vi "MeasureGrowth.vi"(10 "DaysBack":i32=7, 11 "Data":cluster{"Cases":i32[], "Days":timestamp[]}={"Cases"=[0, 0, 0, 0, 2, 2, 2, 2, 2, 3, 3, 3, 6, 6, 6, 6, 6, 6, 6, 6, 7, 7, 8, 8, 8, 8, 8, 8, 8, 8, 10, 10, 10, 10, 10, 10, 11, 11, 12, 12, 21, 25, 35, 51, 59, 102, 116, 167, 179, 247, 250, 305, 372, 480, 588, 741, 892, 1065, 1289, 1524, 1826, 2253, 2641, 3176, 4035, 4863, 5671, 6352, 7412, 8570, 9939, 11170, 12563, 13886], "Days"=[timestamp(3662524800 s since 1904-01-01), timestamp(3662611200 s since 1904-01-01), timestamp(3662697600 s since 1904-01-01), timestamp(3662784000 s since 1904-01-01), timestamp(3662870400 s since 1904-01-01), timestamp(3662956800 s since 1904-01-01), timestamp(3663043200 s since 1904-01-01), timestamp(3663129600 s since 1904-01-01), timestamp(3663216000 s since 1904-01-01), timestamp(3663302400 s since 1904-01-01), timestamp(3663388800 s since 1904-01-01), timestamp(3663475200 s since 1904-01-01), timestamp(3663561600 s since 1904-01-01), timestamp(3663648000 s since 1904-01-01), timestamp(3663734400 s since 1904-01-01), timestamp(3663820800 s since 1904-01-01), timestamp(3663907200 s since 1904-01-01), timestamp(3663993600 s since 1904-01-01), timestamp(3664080000 s since 1904-01-01), timestamp(3664166400 s since 1904-01-01), timestamp(3664252800 s since 1904-01-01), timestamp(3664339200 s since 1904-01-01), timestamp(3664425600 s since 1904-01-01), timestamp(3664512000 s since 1904-01-01), timestamp(3664598400 s since 1904-01-01), timestamp(3664684800 s since 1904-01-01), timestamp(3664771200 s since 1904-01-01), timestamp(3664857600 s since 1904-01-01), timestamp(3664944000 s since 1904-01-01), timestamp(3665030400 s since 1904-01-01), timestamp(3665116800 s since 1904-01-01), timestamp(3665203200 s since 1904-01-01), timestamp(3665289600 s since 1904-01-01), timestamp(3665376000 s since 1904-01-01), timestamp(3665462400 s since 1904-01-01), timestamp(3665548800 s since 1904-01-01), timestamp(3665635200 s since 1904-01-01), timestamp(3665721600 s since 1904-01-01), timestamp(3665808000 s since 1904-01-01), timestamp(3665894400 s since 1904-01-01), timestamp(3665980800 s since 1904-01-01), timestamp(3666067200 s since 1904-01-01), timestamp(3666153600 s since 1904-01-01), timestamp(3666240000 s since 1904-01-01), timestamp(3666326400 s since 1904-01-01), timestamp(3666412800 s since 1904-01-01), timestamp(3666499200 s since 1904-01-01), timestamp(3666585600 s since 1904-01-01), timestamp(3666672000 s since 1904-01-01), timestamp(3666758400 s since 1904-01-01), timestamp(3666844800 s since 1904-01-01), timestamp(3666931200 s since 1904-01-01), timestamp(3667017600 s since 1904-01-01), timestamp(3667104000 s since 1904-01-01), timestamp(3667190400 s since 1904-01-01), timestamp(3667276800 s since 1904-01-01), timestamp(3667363200 s since 1904-01-01), timestamp(3667449600 s since 1904-01-01), timestamp(3667536000 s since 1904-01-01), timestamp(3667622400 s since 1904-01-01), timestamp(3667708800 s since 1904-01-01), timestamp(3667795200 s since 1904-01-01), timestamp(3667881600 s since 1904-01-01), timestamp(3667968000 s since 1904-01-01), timestamp(3668054400 s since 1904-01-01), timestamp(3668140800 s since 1904-01-01), timestamp(3668227200 s since 1904-01-01), timestamp(3668313600 s since 1904-01-01), timestamp(3668400000 s since 1904-01-01), timestamp(3668486400 s since 1904-01-01), timestamp(3668572800 s since 1904-01-01), timestamp(3668659200 s since 1904-01-01), timestamp(3668745600 s since 1904-01-01), timestamp(3668832000 s since 1904-01-01)]}) -> (0 "Plot":T1(graph)=[{"Days"=[timestamp(3662524800 s since 1904-01-01), timestamp(3662611200 s since 1904-01-01), timestamp(3662697600 s since 1904-01-01), timestamp(3662784000 s since 1904-01-01), timestamp(3662870400 s since 1904-01-01), timestamp(3662956800 s since 1904-01-01), timestamp(3663043200 s since 1904-01-01), timestamp(3663129600 s since 1904-01-01), timestamp(3663216000 s since 1904-01-01), timestamp(3663302400 s since 1904-01-01), timestamp(3663388800 s since 1904-01-01), timestamp(3663475200 s since 1904-01-01), timestamp(3663561600 s since 1904-01-01), timestamp(3663648000 s since 1904-01-01), timestamp(3663734400 s since 1904-01-01), timestamp(3663820800 s since 1904-01-01), timestamp(3663907200 s since 1904-01-01), timestamp(3663993600 s since 1904-01-01), timestamp(3664080000 s since 1904-01-01), timestamp(3664166400 s since 1904-01-01), timestamp(3664252800 s since 1904-01-01), timestamp(3664339200 s since 1904-01-01), timestamp(3664425600 s since 1904-01-01), timestamp(3664512000 s since 1904-01-01), timestamp(3664598400 s since 1904-01-01), timestamp(3664684800 s since 1904-01-01), timestamp(3664771200 s since 1904-01-01), timestamp(3664857600 s since 1904-01-01), timestamp(3664944000 s since 1904-01-01), timestamp(3665030400 s since 1904-01-01), timestamp(3665116800 s since 1904-01-01), timestamp(3665203200 s since 1904-01-01), timestamp(3665289600 s since 1904-01-01), timestamp(3665376000 s since 1904-01-01), timestamp(3665462400 s since 1904-01-01), timestamp(3665548800 s since 1904-01-01), timestamp(3665635200 s since 1904-01-01), timestamp(3665721600 s since 1904-01-01), timestamp(3665808000 s since 1904-01-01), timestamp(3665894400 s since 1904-01-01), timestamp(3665980800 s since 1904-01-01), timestamp(3666067200 s since 1904-01-01), timestamp(3666153600 s since 1904-01-01), timestamp(3666240000 s since 1904-01-01), timestamp(3666326400 s since 1904-01-01), timestamp(3666412800 s since 1904-01-01), timestamp(3666499200 s since 1904-01-01), timestamp(3666585600 s since 1904-01-01), timestamp(3666672000 s since 1904-01-01), timestamp(3666758400 s since 1904-01-01), timestamp(3666844800 s since 1904-01-01), timestamp(3666931200 s since 1904-01-01), timestamp(3667017600 s since 1904-01-01), timestamp(3667104000 s since 1904-01-01), timestamp(3667190400 s since 1904-01-01), timestamp(3667276800 s since 1904-01-01), timestamp(3667363200 s since 1904-01-01), timestamp(3667449600 s since 1904-01-01), timestamp(3667536000 s since 1904-01-01), timestamp(3667622400 s since 1904-01-01), timestamp(3667708800 s since 1904-01-01), timestamp(3667795200 s since 1904-01-01), timestamp(3667881600 s since 1904-01-01), timestamp(3667968000 s since 1904-01-01), timestamp(3668054400 s since 1904-01-01), timestamp(3668140800 s since 1904-01-01), timestamp(3668227200 s since 1904-01-01), timestamp(3668313600 s since 1904-01-01), timestamp(3668400000 s since 1904-01-01), timestamp(3668486400 s since 1904-01-01), timestamp(3668572800 s since 1904-01-01), timestamp(3668659200 s since 1904-01-01), timestamp(3668745600 s since 1904-01-01), timestamp(3668832000 s since 1904-01-01)], "ConfirmedCases"=[0.0, 0.0, 0.0, 0.0, 0.0, 0.0, 0.0, 0.0, 0.0, 0.0, 0.0, 0.0, 0.0, 0.0, 0.0, 0.0, 0.0, 0.0, 0.0, 0.0, 0.0, 0.0, 0.0, 0.0, 0.0, 0.0, 0.0, 0.0, 0.0, 0.0, 0.0, 0.0, 0.0, 0.0, 0.0, 0.0, 0.0, 0.0, 0.0, 0.0, 0.0, 0.0, 1.0, 1.0, 1.0, 1.0, 1.0, 2.0, 3.0, 4.0, 4.0, 4.0, 4.0, 6.0, 11.0, 14.0, 17.0, 19.0, 24.0, 29.0, 33.0, 40.0, 52.0, 67.0, 83.0, 100.0, 121.0, 132.0, 149.0, 182.0, 212.0, 243.0, 282.0, 321.0]}, {"Days"=[timestamp(3668313600 s since 1904-01-01), timestamp(3668400000 s since 1904-01-01), timestamp(3668486400 s since 1904-01-01), timestamp(3668572800 s since 1904-01-01), timestamp(3668659200 s since 1904-01-01), timestamp(3668745600 s since 1904-01-01), timestamp(3668832000 s since 1904-01-01)], "ConfirmedCases"=[132.01823524302534, 153.55263572024907, 178.59966006386384, 207.73227646213113, 241.6169138771523, 281.0287070731711, 326.8692283660796]}, {"Days"=[timestamp(3668313600 s since 1904-01-01), timestamp(3668400000 s since 1904-01-01), timestamp(3668486400 s since 1904-01-01), timestamp(3668572800 s since 1904-01-01), timestamp(3668659200 s since 1904-01-01), timestamp(3668745600 s since 1904-01-01), timestamp(3668832000 s since 1904-01-01)], "ConfirmedCases"=[140.59609548662908, 162.8828644131387, 188.9766356577397, 219.6124606618654, 255.65531024069676, 298.10468948116306, 348.1074955925532]}, {"Days"=[timestamp(3668313600 s since 1904-01-01), timestamp(3668400000 s since 1904-01-01), timestamp(3668486400 s since 1904-01-01), timestamp(3668572800 s since 1904-01-01), timestamp(3668659200 s since 1904-01-01), timestamp(3668745600 s since 1904-01-01), timestamp(3668832000 s since 1904-01-01)], "ConfirmedCases"=[123.96371589380509, 144.75685960943596, 168.7924989452066, 196.49476425010758, 228.34938580605382, 264.9308682016178, 306.9267217896756]}, {"Days"=[timestamp(3668313600 s since 1904-01-01), timestamp(3668400000 s since 1904-01-01), timestamp(3668486400 s since 1904-01-01), timestamp(3668572800 s since 1904-01-01), timestamp(3668659200 s since 1904-01-01), timestamp(3668745600 s since 1904-01-01), timestamp(3668832000 s since 1904-01-01)], "ConfirmedCases"=[140.59609548662908, 160.133980854025, 182.38694136848164, 207.73227646213113, 236.5997168457177, 269.47871060219524, 306.9267217896756]}, {"Days"=[timestamp(3668313600 s since 1904-01-01), timestamp(3668400000 s since 1904-01-01), timestamp(3668486400 s since 1904-01-01), timestamp(3668572800 s since 1904-01-01), timestamp(3668659200 s since 1904-01-01), timestamp(3668745600 s since 1904-01-01), timestamp(3668832000 s since 1904-01-01)], "ConfirmedCases"=[123.96371589380509, 147.24177723483396, 174.89102199747728, 207.73227646213113, 246.7405026929383, 293.0737423477007, 348.1074955925532]}], 1 "Interval":dbl, 2 "PlusMinus":dbl=2.4408305776857144, 3 "Growth":dbl=16.31168636482856, 4 "GrowthLower":dbl=13.896463696073248, 6 "GrowthUpper":dbl=18.778124851444677)   [LabVIEW 2017]
uses:
  <vilib>/Analysis/6fits.llb/Prediction Interval (Linear).vi
  <vilib>/Analysis/1siggen.llb/Ramp Pattern by Samples.vi
  <vilib>/Analysis/NI_AALPro.lvlib
  <vilib>/Analysis/NI_AALBase.lvlib
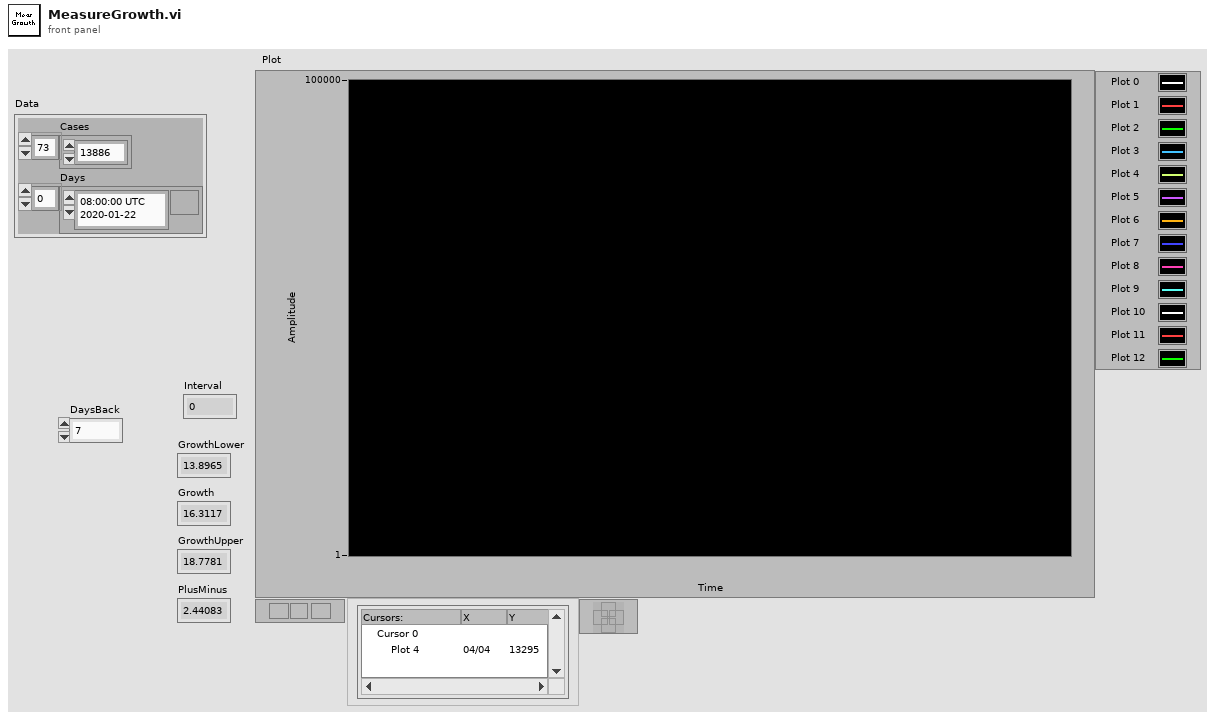
[diagram p1: front panel]
types:
  T1 = cluster{"Days":timestamp[], "ConfirmedCases":dbl[]}[]
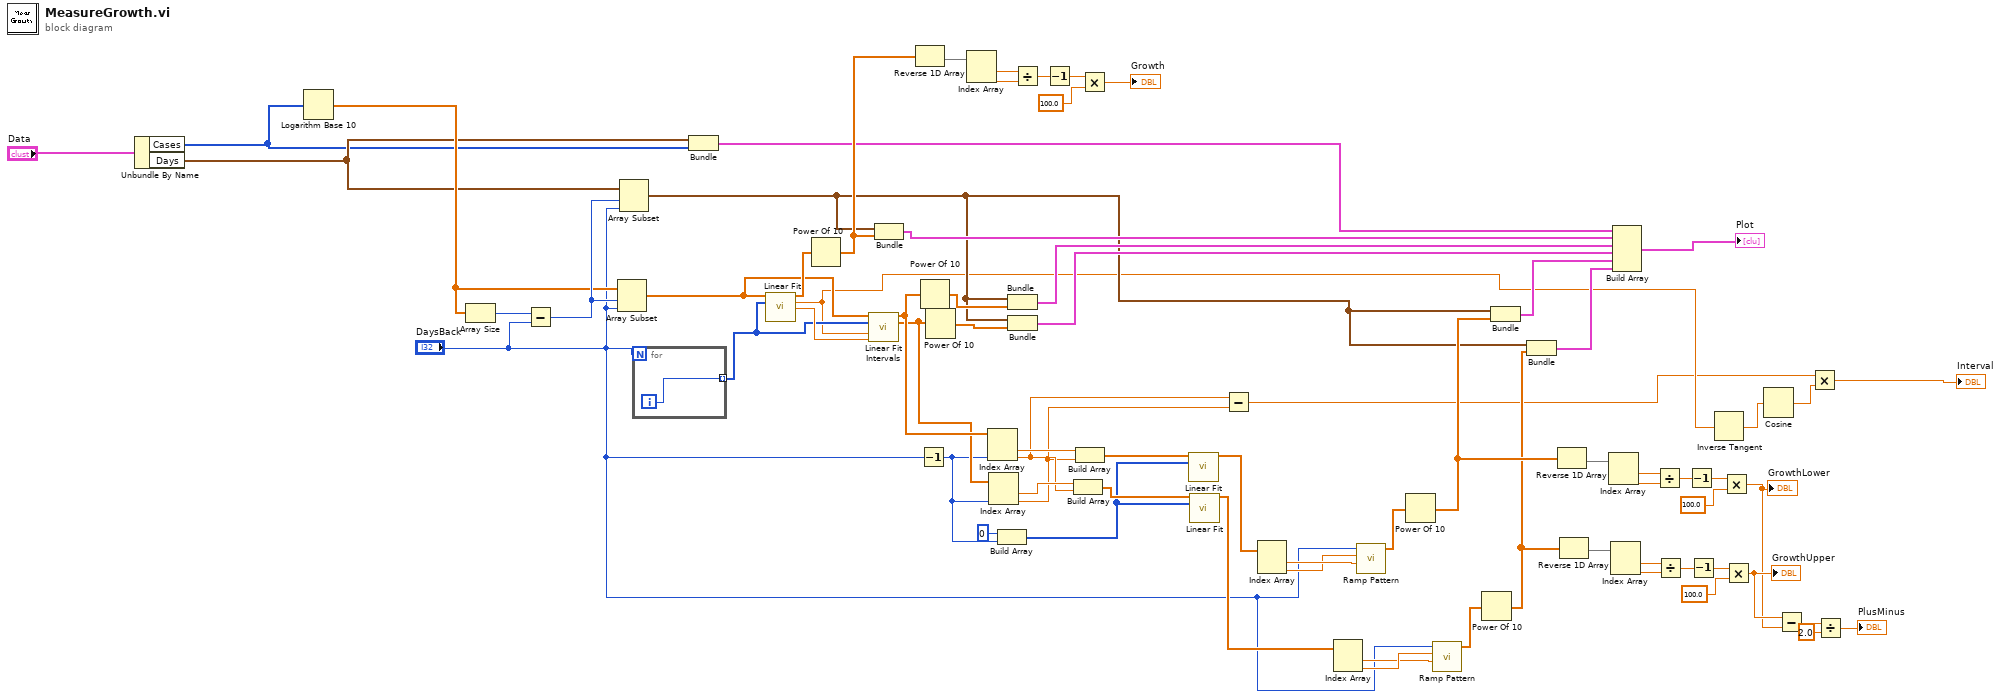
[diagram p0: block diagram]
diagram:
  n1 = Unbundle By Name("Data") -> ("Cases"=w8:i32[], "Days"=w16:timestamp[])
  n2 = Logarithm Base 10(1:w8) -> (0:w66:dbl[])
  n3 = Array Size(array=w66) -> (size(s)=w72:i32)
  n4 = Subtract(x=w72, y="DaysBack") -> (x-y=w71:i32)
  n5 = Array Subset(array=w66, index=w71, length="DaysBack") -> (w19:dbl[])
  n6 = Array Subset(array=w16, index=w71, length="DaysBack") -> (w15:timestamp[])
  n7 = for {
    N: "DaysBack" -> [_]
    tunnel: [w73] -> w18 mode=indexing
    i -> [w73]
  }
  n8 = Bundle("Days"=w16, "Cases"=w8) -> (w17:cluster{"Days":timestamp[], "Cases":i32[]})  [unwired: 1 in]
  n9 = call <vilib>:"Linear Fit.vi"("Y"=w19, "X"=w18) -> ("Best Linear Fit"=w65:dbl[], "slope"=w4:dbl, "intercept"=w69:dbl)  [unwired: 9 in, 2 out]
  n10 = Power Of 10(x=w65) -> (10^x=w63:dbl[])
  n11 = call-poly <vilib>:"Linear Fit Intervals.vi"("Y"=w19, "X"=w18, "slope"=w4, "intercept"=w69) -> ("Upper Bound"=w50:dbl[], "Lower Bound"=w49:dbl[])  [unwired: 9 in, 1 out]
  n12 = Bundle(w15, w63) -> (w70:cluster{timestamp[], dbl[]})  [unwired: 1 in]
  n13 = Reverse 1D Array(array=w63) -> (reversed array=w62:dbl[])
  n14 = Decrement(x="DaysBack") -> (x-1=w48:i32)
  n15 = Power Of 10(x=w50) -> (10^x=w54:dbl[])
  n16 = Power Of 10(x=w49) -> (10^x=w55:dbl[])
  n17 = Index Array(array=w62) -> (element #1=w61:dbl, element #2=w60:dbl)  [unwired: 2 in]
  n18 = Index Array(array=w50, index #2=w48) -> (element #1=w52:dbl, element #2=w3:dbl)  [unwired: 1 in]
  n19 = Index Array(array=w49, index #2=w48) -> (element #1=w45:dbl, element #2=w2:dbl)  [unwired: 1 in]
  n20 = Build Array(0 ("element"), w48) -> (w46:i32[])
  n21 = Bundle(w15, w54) -> (w68:cluster{timestamp[], dbl[]})  [unwired: 1 in]
  n22 = Bundle(w15, w55) -> (w67:cluster{timestamp[], dbl[]})  [unwired: 1 in]
  n23 = Divide(x=w61, y=w60) -> (x/y=w59:dbl)
  n24 = Decrement(x=w59) -> (x-1=w58:dbl)
  n25 = Build Array(w45, w3) -> (w47:dbl[])
  n26 = Build Array(w52, w2) -> (w51:dbl[])
  n27 = Multiply(x=w58, y=100.0) -> (x*y=→"Growth":dbl)
  n28 = call <vilib>:"Linear Fit.vi"("Y"=w51, "X"=w46) -> ("Best Linear Fit"=w44:dbl[])  [unwired: 9 in, 4 out]
  n29 = call <vilib>:"Linear Fit.vi"("Y"=w47, "X"=w46) -> ("Best Linear Fit"=w37:dbl[])  [unwired: 9 in, 4 out]
  n30 = Subtract(x=w3, y=w2) -> (x-y=w1:dbl)
  n31 = Index Array(array=w44) -> (element #1=w43:dbl, element #2=w42:dbl)  [unwired: 2 in]
  n32 = Index Array(array=w37) -> (element #1=w38:dbl, element #2=w39:dbl)  [unwired: 2 in]
  n33 = call-poly <vilib>:"Ramp Pattern.vi"("start"=w43, "end"=w42, "samples"="DaysBack") -> ("Ramp Pattern"=w41:dbl[])  [unwired: 7 in, 1 out]
  n34 = Power Of 10(x=w41) -> (10^x=w27:dbl[])
  n35 = call-poly <vilib>:"Ramp Pattern.vi"("start"=w38, "end"=w39, "samples"="DaysBack") -> ("Ramp Pattern"=w40:dbl[])  [unwired: 7 in, 1 out]
  n36 = Power Of 10(x=w40) -> (10^x=w20:dbl[])
  n37 = Bundle(w15, w27) -> (w35:cluster{timestamp[], dbl[]})  [unwired: 1 in]
  n38 = Bundle(w15, w20) -> (w34:cluster{timestamp[], dbl[]})  [unwired: 1 in]
  n39 = Reverse 1D Array(array=w27) -> (reversed array=w28:dbl[])
  n40 = Reverse 1D Array(array=w20) -> (reversed array=w26:dbl[])
  n41 = Index Array(array=w28) -> (element #1=w29:dbl, element #2=w30:dbl)  [unwired: 2 in]
  n42 = Index Array(array=w26) -> (element #1=w25:dbl, element #2=w24:dbl)  [unwired: 2 in]
  n43 = Build Array(w17, w70, w68, w67, w35, w34) -> (→"Plot":cluster{"Days":timestamp[], "Cases":dbl[]}[])
  n44 = Divide(x=w29, y=w30) -> (x/y=w31:dbl)
  n45 = Divide(x=w25, y=w24) -> (x/y=w23:dbl)
  n46 = Decrement(x=w31) -> (x-1=w32:dbl)
  n47 = Decrement(x=w23) -> (x-1=w22:dbl)
  n48 = Inverse Tangent(1:w4) -> (0:w7:dbl)
  n49 = Multiply(x=w32, y=100.0) -> (x*y=w13:dbl)
  "GrowthLower" <- w13
  n50 = Multiply(x=w22, y=100.0) -> (x*y=w14:dbl)
  "GrowthUpper" <- w14
  n51 = Cosine(x=w7) -> (cos(x)=w6:dbl)
  n52 = Subtract(x=w14, y=w13) -> (x-y=w12:dbl)
  n53 = Multiply(x=w1, y=w6) -> (x*y=→"Interval":dbl)
  n54 = Divide(x=w12, y=2.0) -> (x/y=→"PlusMinus":dbl)
